vi "Write gen for DF.vi"(8 "error in (no error)":errorcluster, 9 "use arb files":bool=TRUE, 10 "gen for DF":bool, 11 "device_type in":refnum<class "device_type.lvclass">) -> (0 "error out":errorcluster, 3 "device_type out":refnum<class "device_type.lvclass">)   [LabVIEW 2021, in "device_type.lvclass"]
uses:
  device_type.lvclass
  device_type.lvclass/device_type.ctl
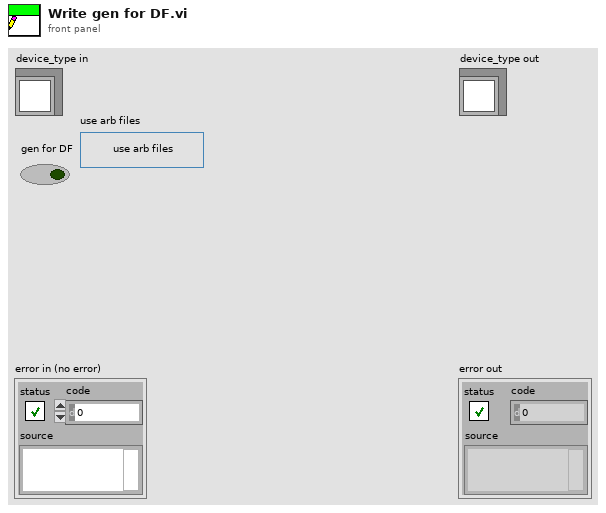
[diagram p1: front panel]
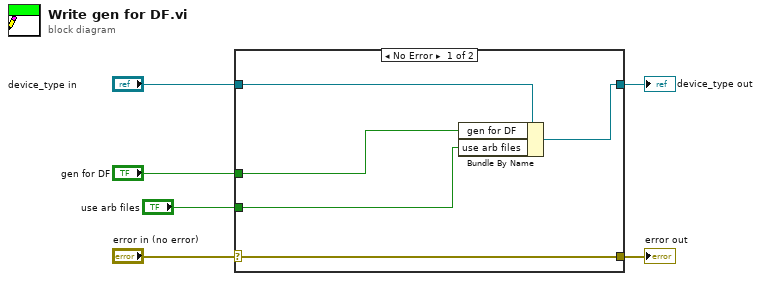
[diagram p0: block diagram]
diagram:
  n1 = case shown="No Error" "error in (no error)" {
    selector: "error in (no error)" -> [w11 w12]
    tunnel: [w11 w12] -> w5
    tunnel: [w9 w13] -> w3
    tunnel: "device_type in" -> [w10 w13]
    tunnel: "gen for DF" -> [w8 _]
    tunnel: "use arb files" -> [w7 _]
    frame No Error {
      n2 = Bundle By Name(cluster=w10, "gen for DF"=w8, "use arb files"=w7) -> (w9:refnum<class "device_type.lvclass">)
    }
    frame Error {
    }
  }
  "error out" <- w5
  "device_type out" <- w3
